vi "HEWH Check Temp Spec.vi"(6 "Cold Water Gallons":dbl[](array[numeric]), 8 "error in (no error)":errorcluster, 10 "RTD IN Full Data Set (Each Draw)":dbl[](array[numeric])) -> (0 "error out":errorcluster, 2 "Draw Temp In Spec?":bool, 3 "Data Array":dbl[](array[numeric]))   [LabVIEW 2023]
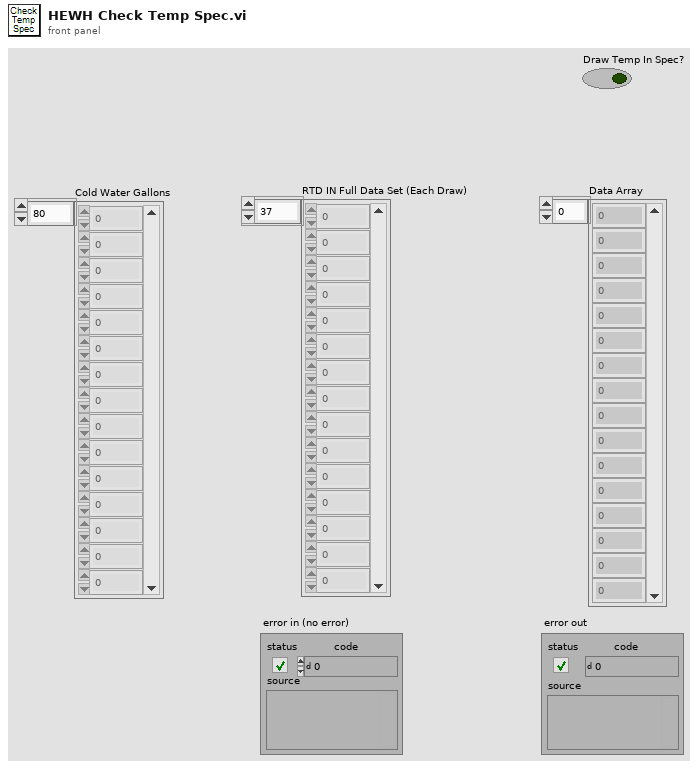
[diagram p1: front panel]
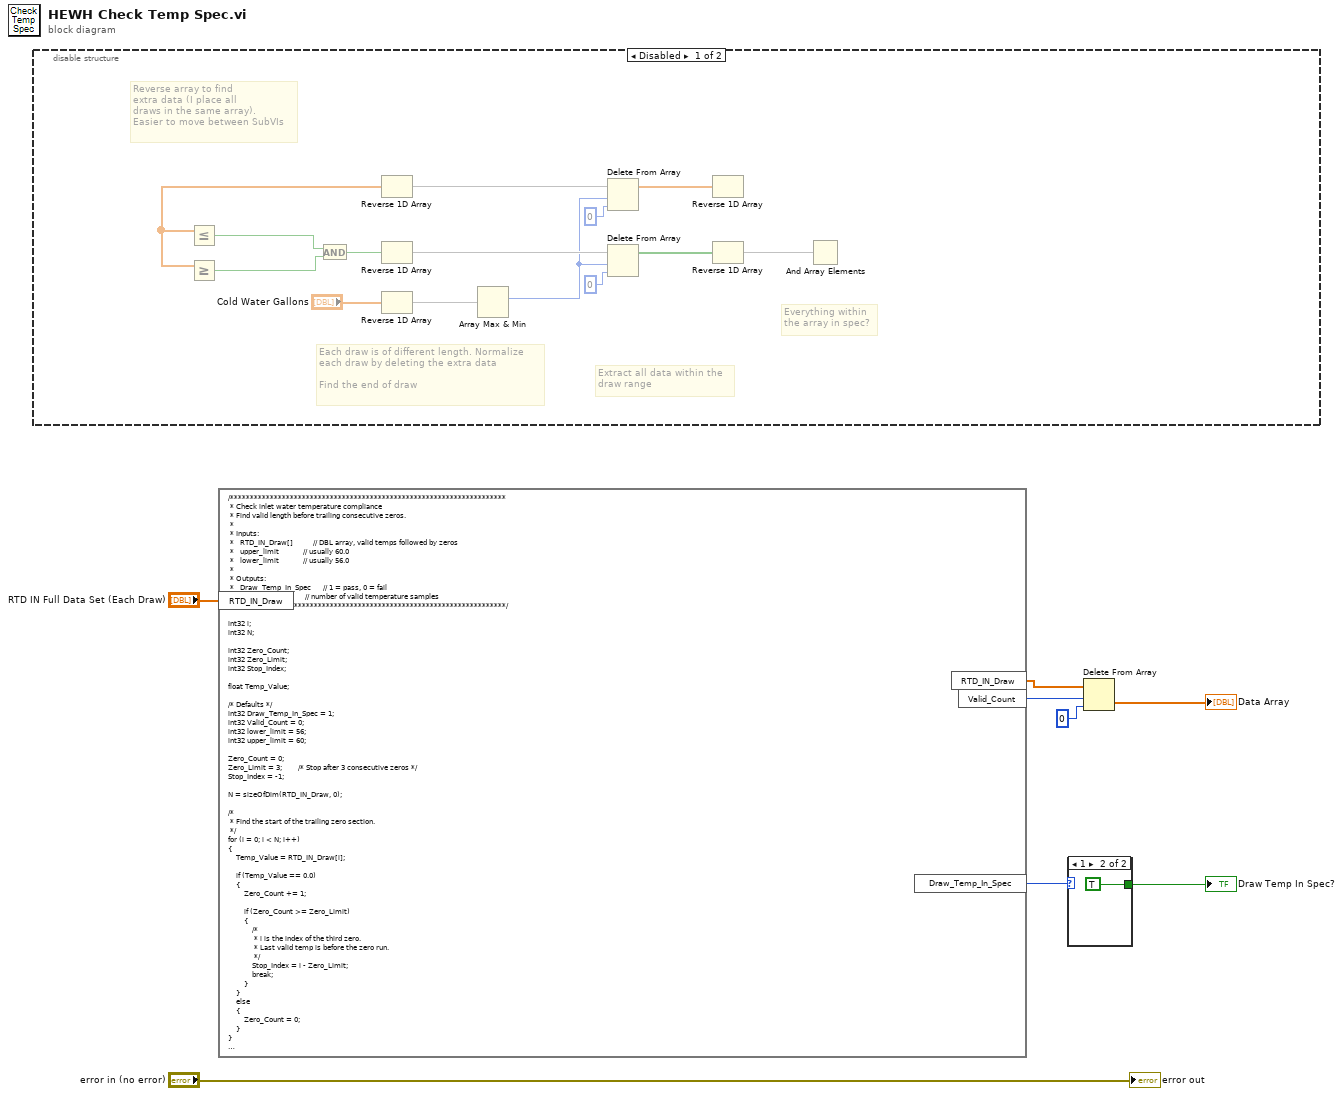
[diagram p0: block diagram]
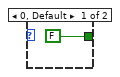
[diagram p3: hidden frame]
diagram:
  n1 = disable-structure shown="Disabled" {
    frame Disabled {
      # "Extract all data within the \ndraw range"
      # "Reverse array to find\nextra data (I place all\ndraws in the same array). \nEasier to move between SubVIs"
      # "Each draw is of different length. Normalize\neach draw by deleting the extra data\n\nFind the end of draw"
      # "Everything within\nthe array in spec?"
      n2 = Reverse 1D Array() -> (array=w9:ext[], reversed array=w17:ext[])
      n3 = Less Or Equal?(x=w9) -> (x <= y?=w12:bool)  [unwired: 1 in]
      n4 = Greater Or Equal?(x=w9) -> (x >= y?=w11:bool)  [unwired: 1 in]
      n5 = And(x=w12, y=w11) -> (x .and. y?=w10:bool)
      n6 = Reverse 1D Array(array=w10) -> (reversed array=w16:bool[])
      n7 = Reverse 1D Array(array="Cold Water Gallons") -> (reversed array=w14:dbl[])
      n8 = Array Max & Min(array=w14) -> (max index (indices)=w13:i32)  [unwired: 3 out]
      n9 = Delete From Array "Delete From Array"(array=w17, length=w13, index=0) -> (array with subset deleted=w18:ext[])  [unwired: 1 out]
      n10 = Delete From Array "Delete From Array"(array=w16, length=w13, index=0) -> (array with subset deleted=w21:bool[])  [unwired: 1 out]
      n11 = Reverse 1D Array(array=w18) -> ()  [unwired: 1 out]
      n12 = Reverse 1D Array(array=w21) -> (reversed array=w22:bool[])
      n13 = And Array Elements(Boolean array=w22) -> ()  [unwired: 1 out]
    }
    frame Enabled {
    }
  }
  n14 = formula code="/*********************************************************************\n * Check inlet water temperature compliance\n * Find valid length before trailing consecutive zeros.\n *\n * Inputs:\n *   RTD_IN_Draw[]          // DBL array, valid temps followed by zeros\n *   upper_limit            // usually 60.0\n *   lower_limit            // usually 56.0\n *\n * Outputs:\n *   Draw_Temp_In_Spec      // 1 = pass, 0 = fail\n *   Valid_Count            // number of valid temperature samples\n *********************************************************************/\n\nint32 i;\nint32 N;\n\nint32 Zero_Count;\nint32 Zero_Limit;\nint32 Stop_Index;\n\nfloat Temp_Value;\n\n/* Defaults */\nint32 Draw_Temp_In_Spec = 1;\nint32 Valid_Count = 0;\nint32 lower_limit = 56;\nint32 upper_limit = 60;\n\nZero_Count = 0;\nZero_Limit = 3;        /* Stop after 3 consecutive zeros */\nStop_Index = -1;\n\nN = sizeOfDim(RTD_IN_Draw, 0);\n\n/*\n * Find the start of the trailing zero section.\n */\nfor (i = 0; i < N; i++)\n{\n    Temp_Value = RTD_IN_Draw[i];\n\n    if (Temp_Value == 0.0)\n    {\n        Zero_Count += 1;\n\n        if (Zero_Count >= Zero_Limit)\n        {\n            /*\n             * i is the index of the third zero.\n             * Last valid temp is before the zero run.\n             */\n            Stop_Index = i - Zero_Limit;\n            break;\n        }\n    }\n    else\n    {\n        Zero_Count = 0;\n    }\n}\n\n/*\n * If no trailing zero section was found, use the full array.\n */\nif (Stop_Index < 0)\n{\n    Stop_Index = N - 1;\n}\n\n/*\n * Number of valid samples to keep.\n */\nValid_Count = Stop_Index + 1;\n\n/*\n * Check only the valid temperature samples.\n */\nif (Valid_Count > 0)\n{\n    for (i = 0; i < Valid_Count; i++)\n    {\n        Temp_Value = RTD_IN_Draw[i];\n\n        if (Temp_Value < lower_limit || Temp_Value > upper_limit)\n        {\n            Draw_Temp_In_Spec = 0;\n        }\n    }\n}\nelse\n{\n    Draw_Temp_In_Spec = 0;\n}"("RTD_IN_Draw"="RTD IN Full Data Set (Each Draw)") -> ("RTD_IN_Draw"=w6:dbl[], "Draw_Temp_In_Spec"=w5:i32, "Valid_Count"=w3:i32)
  n15 = case shown="1" w5 {
    tunnel: [FALSE TRUE] -> w1
    frame 0, Default {
    }
    frame 1 {
    }
  }
  "Draw Temp In Spec?" <- w1
  n16 = Delete From Array "Delete From Array"(array=w6, length=w3, index=0) -> (deleted portion=→"Data Array":dbl[])  [unwired: 1 out]
  "error out" <- "error in (no error)"
